vi "Create Workbook.vi"() -> (0 "error out":errorcluster, 3 "hssfworkbook":refnum<k24>)   [LabVIEW 2013]
uses:
  C:/PhaeronGit/LVNPOI/Resources/NPOI 2.1.1 dotnet2/NPOI.dll
  Resources/NPOI 2.1.1 dotnet2/NPOI.dll
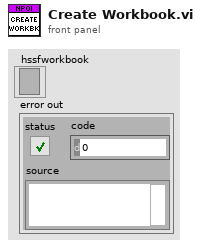
[diagram p1: front panel]
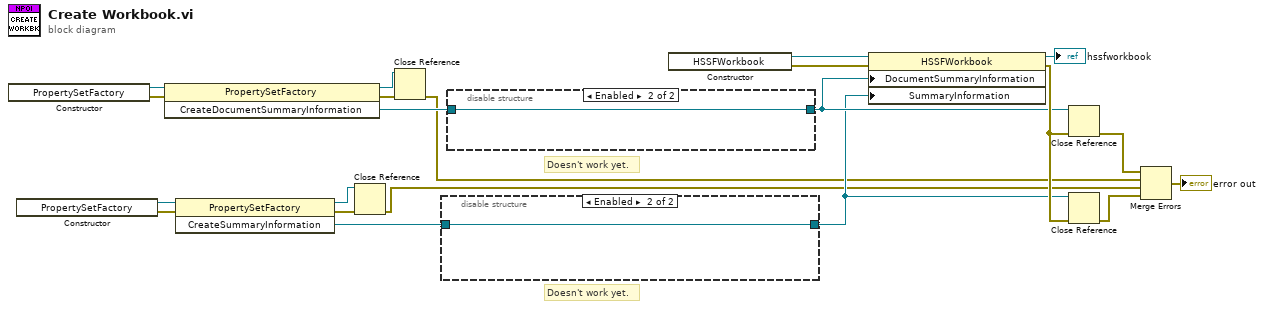
[diagram p0: block diagram]
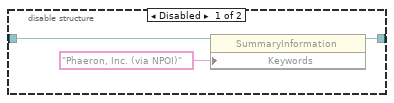
[diagram p2: hidden frame]
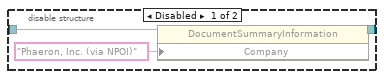
[diagram p3: hidden frame]
diagram:
  # "Doesn't work yet."
  # "Doesn't work yet."
  n1 = constructor class="PropertySetFactory"() -> (reference out=w19:refnum<k24>, error out=w18:errorcluster)  [unwired: 3 in, 1 out]
  n2 = constructor class="PropertySetFactory"() -> (reference out=w11:refnum<k24>, error out=w12:errorcluster)  [unwired: 3 in, 1 out]
  n3 = invoke class="PropertySetFactory" method="CreateDocumentSummaryInformation"(reference=w19, error in=w18) -> (reference out=w15:refnum<k24>, error out=w16:errorcluster, "CreateDocumentSummaryInformation"=w17:refnum<k24>)  [unwired: 1 in]
  n4 = invoke class="PropertySetFactory" method="CreateSummaryInformation"(reference=w11, error in=w12) -> (reference out=w10:refnum<k24>, error out=w14:errorcluster, "CreateSummaryInformation"=w13:refnum<k24>)  [unwired: 1 in]
  n5 = Close Reference(reference=w10, error in (no error)=w14) -> (error out=w3:errorcluster)
  n6 = Close Reference(reference=w15, error in (no error)=w16) -> (error out=w4:errorcluster)
  n7 = disable-structure shown="Enabled" {
    disable-tunnel: w13 -> [w24 w25]
    disable-tunnel: [w22 w25] -> w7
    frame Disabled {
      n8 = property class="SummaryInformation"(reference=w24, "Keywords"="Phaeron, Inc. (via NPOI)" ("Company")) -> (reference out=w22:refnum<k24>)  [unwired: 1 in, 1 out]
    }
    frame Enabled {
    }
  }
  n9 = disable-structure shown="Enabled" {
    disable-tunnel: w17 -> [w28 w29]
    disable-tunnel: [w26 w29] -> w8
    frame Disabled {
      n10 = property class="DocumentSummaryInformation"(reference=w28, "Company"="Phaeron, Inc. (via NPOI)") -> (reference out=w26:refnum<k24>)  [unwired: 1 in, 1 out]
    }
    frame Enabled {
    }
  }
  n11 = constructor class="HSSFWorkbook"() -> (reference out=w21:refnum<k24>, error out=w20:errorcluster)  [unwired: 3 in, 1 out]
  n12 = property class="HSSFWorkbook"(reference=w21, error in=w20, "DocumentSummaryInformation"=w8, "SummaryInformation"=w7) -> (reference out=→"hssfworkbook":refnum<k24>, error out=w9:errorcluster)
  n13 = Close Reference(reference=w8, error in (no error)=w9) -> (error out=w5:errorcluster)
  n14 = Close Reference(reference=w7, error in (no error)=w9) -> (error out=w2:errorcluster)
  n15 = Merge Errors(w5, w4, w3, w2) -> (→"error out":errorcluster)
